vi "KE236_CommandsGlobal.vi"() -> ()   [LabVIEW 2019, in "KE236.lvclass"]
uses:
  KE236.lvclass
panel:
  in  "Keithley 236 GPIB Setup":T1={"Instrument name"="Keithley 236", "Command \"Reset\""="J0X", "Command \"Initialise\""="K0Y0G4,2,0N0R1O0T4,1,0,0F0,0P3S2B0,0,0L%1.6f,%dH0X", "Command \"Arm\""="B0,0,0N1X", "Command \"SetVolts\""="B%3.2f,0,0F0,0H0X", "Command \"Compliance?\""="U3X", "Command \"Standby\""="B0,0,0N0X", "Command \"Read Current\""="H0X"}
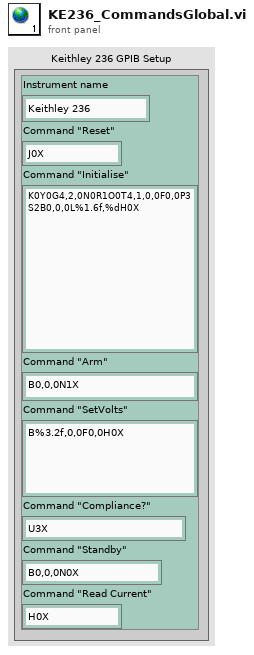
[diagram p1: front panel]
types:
  T1 = cluster{"Instrument name":string, "Command \"Reset\"":string, "Command \"Initialise\"":string, "Command \"Arm\"":string, "Command \"SetVolts\"":string, "Command \"Compliance?\"":string, "Command \"Standby\"":string, "Command \"Read Current\"":string}
diagram:
